vi "PythonName.vi"(6 "add self":bool, 8 "error in":errorcluster, 11 "Node in":refnum<class "Node.lvclass">) -> (0 "error out":errorcluster, 3 "Node out":refnum<class "Node.lvclass">, 5 "name":string, 7 "UID":string)   [LabVIEW 2014, in "Raspberry Pi Compatible Compiler for LabVIEW.lvlib" / "Node.lvclass"]
uses:
  Node.lvclass
  Python/Parsing/Python Functions.lvlib
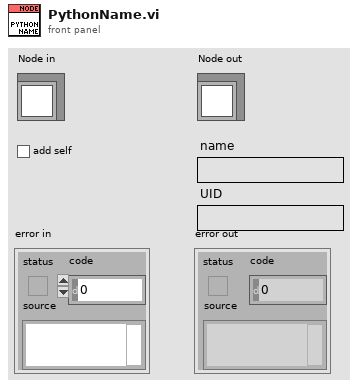
[diagram p1: front panel]
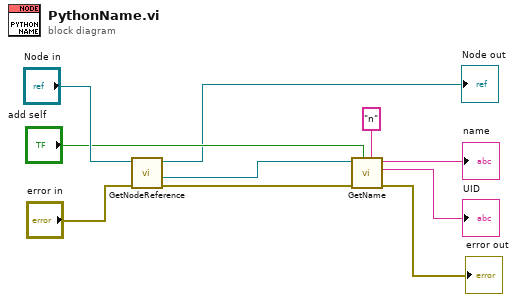
[diagram p0: block diagram]
diagram:
  n1 = call "GetNodeReference.vi"("error in"="error in", "Node in"="Node in") -> ("error out"=w4:errorcluster, "reference out"=w8:refnum<vi>, "Node out"=→"Node out":refnum<class "Node.lvclass">)  [unwired: 7 in]
  n2 = call "GetName.vi"("base name"="n", "add self"="add self", "error in"=w4, "GObj Refnum"=w8) -> ("error out"=→"error out":errorcluster, "UID"=→"UID":string, "name"=→"name":string)  [unwired: 5 in]
